vi "Swerve_Slave.vi"(4 "Intended Angle":i32, 5 "PortIn":i32) -> ()   [LabVIEW 2012]
uses:
  <vilib>/NXT/Block Support/NXT_OutputPort.ctl
  <vilib>/NXT/Dual Mode Library/Motors/Rotation.vi
  <vilib>/NXT/Dual Mode Library/prims/inRangeAndCoerce/inRangeAndCoerce_float.vi
  <vilib>/NXT/NXTIO Xnodes/NXTIONodeSubVIs/NXTMoveMotors.vi
  <vilib>/NXT/NXTIO Xnodes/NXTIONodeSubVIs/NXTStopMotors.vi
  <vilib>/NXT/NXTIO Xnodes/AddressXNode/NXTIOAddress.xnode
  <vilib>/NXT/Subs/LVHSConnector.ctl
  <vilib>/NXT/NXTIO Xnodes/NXTIOXNode/NXTIO.xnode
  <vilib>/NXT/LegoClasses/BrickReference/BrickReference.lvclass
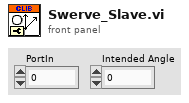
[diagram p1: front panel]
types:
  T1 = typedef "NXT_OutputPort.ctl" = u8
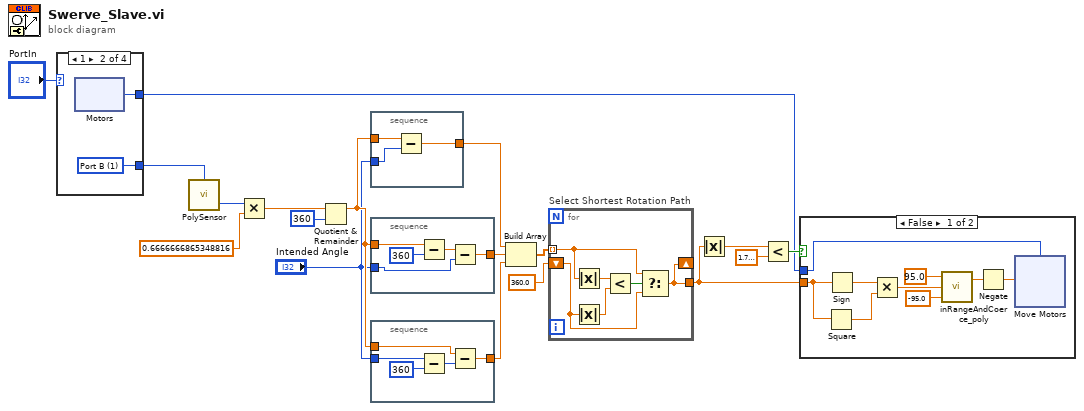
[diagram p0: block diagram]
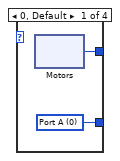
[diagram p2: hidden frame]
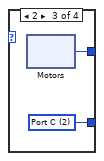
[diagram p3: hidden frame]
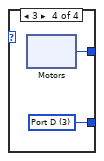
[diagram p4: hidden frame]
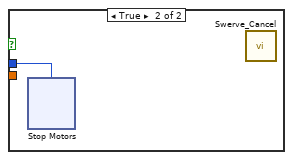
[diagram p5: hidden frame]
diagram:
  n1 = case shown="1" "PortIn" {
    tunnel: [w20 w23 w26 w29] -> w2
    tunnel: [w19 w22 w25 w28] -> w1
    frame 0, Default {
      w19 = 0 items=["Port A", "Port B", "Port C", "Port D"] ("Port (Port A)")
      n2 = xnode "Motors"() -> ("Motor"=w20:T1)
    }
    frame 1 {
      w22 = 1 items=["Port A", "Port B", "Port C", "Port D"] ("Port (Port A)")
      n3 = xnode "Motors"() -> ("Motor"=w23:T1)
    }
    frame 2 {
      w25 = 2 items=["Port A", "Port B", "Port C", "Port D"] ("Port (Port A)")
      n4 = xnode "Motors"() -> ("Motor"=w26:T1)
    }
    frame 3 {
      w28 = 3 items=["Port A", "Port B", "Port C", "Port D"] ("Port (Port A)")
      n5 = xnode "Motors"() -> ("Motor"=w29:T1)
    }
  }
  n6 = call-poly <vilib>:"PolySensor.vi"("Port (Port A)"=w1) -> ("Angle of Rotation"=w15:i32)  [unwired: 2 in, 1 out]
  n7 = Multiply(x=w15, y=sgl 0.6666667) -> (x*y=w17:sgl)
  n8 = Quotient & Remainder(x=w17, y=360) -> (x-y*floor(x/y)=w10:sgl)  [unwired: 1 out]
  n9 = stacked-sequence {
    tunnel: w10 -> [w33]
    tunnel: "Intended Angle" -> [w32]
    tunnel: [w31] -> w13
    frame #0 {
      n10 = Subtract(x=w33, y=w32) -> (x-y=w31:sgl)
    }
  }
  n11 = stacked-sequence {
    tunnel: w10 -> [w37]
    tunnel: "Intended Angle" -> [w35]
    tunnel: [w34] -> w12
    frame #0 {
      n12 = Subtract(x=w37, y=360) -> (x-y=w36:sgl)
      n13 = Subtract(x=w36, y=w35) -> (x-y=w34:sgl)
    }
  }
  n14 = stacked-sequence {
    tunnel: w10 -> [w39]
    tunnel: "Intended Angle" -> [w41]
    tunnel: [w42] -> w8
    frame #0 {
      n15 = Subtract(x=w41, y=360) -> (x-y=w40:i32)
      n16 = Subtract(x=w39, y=w40) -> (x-y=w42:sgl)
    }
  }
  n17 = Build Array(w13, w12, w8) -> (w14:sgl[])
  n18 = for "Select Shortest Rotation Path" {
    tunnel: w14 -> [w47] mode=indexing
    shift-right: [w44] -> _
    shift-left: sgl 360.0 ("y") -> [w46]
    tunnel: [w44] -> w5
    n19 = Absolute Value(x=w47) -> (abs(x)=w48:sgl)
    n20 = Absolute Value(x=w46) -> (abs(x)=w45:sgl)
    n21 = Less?(x=w48, y=w45) -> (x < y?=w49:bool)
    n22 = Select(t=w47, s=w49, f=w46) -> (s? t:f=w44:sgl)
  }
  n23 = Absolute Value(x=w5) -> (abs(x)=w4:sgl)
  n24 = Less?(x=w4, y=sgl 1.7) -> (x < y?=w6:bool)
  n25 = case shown="False" w6 {
    tunnel: w5 -> [w53 _]
    tunnel: w2 -> [w55 w66]
    frame False {
      n26 = Square(x=w53) -> (x^2=w51:sgl)
      n27 = Sign(1:w53) -> (0:w52:sgl)
      n28 = Multiply(x=w52, y=w51) -> (x*y=w50:sgl)
      n29 = call-poly <vilib>:"inRangeAndCoerce_poly.vi"("lower limit"=sgl -95.0, "x"=w50, "upper limit"=sgl 95.0) -> ("coerced(x)"=w56:sgl)  [unwired: 1 out]
      n30 = Negate(x=w56) -> (-x=w54:sgl)
      n31 = xnode "Move Motors"("Power/Speed 1"=w54, "Motors"=w55) -> ()  [unwired: 1 in, 1 out]
    }
    frame True {
      n32 = xnode "Stop Motors"("Motors"=w66) -> ()  [unwired: 1 in, 1 out]
      n33 = call "Swerve_Cancel.vi"() -> ()  [unwired: 12 in]
    }
  }
